vi "选择结构（成绩分类）.vi"() -> ()   [LabVIEW 2017]
panel:
  out "c成绩":string="成绩无效！！!"
  in  "分数":dbl
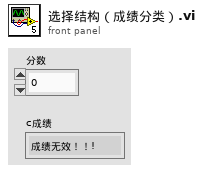
[diagram p1: front panel]
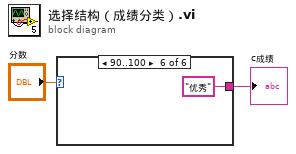
[diagram p0: block diagram]
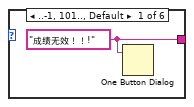
[diagram p2: hidden frame]
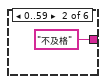
[diagram p3: hidden frame]
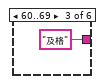
[diagram p4: hidden frame]
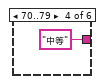
[diagram p5: hidden frame]
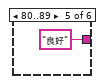
[diagram p6: hidden frame]
diagram:
  n1 = case shown="90..100" "分数" {
    tunnel: [w3 "不及格" ("消息") "及格" ("消息") "中等" ("消息") "良好" ("消息") "优秀" ("消息")] -> w1
    frame ..-1, 101.., Default {
      w3 = "成绩无效！！!" ("消息")
      n2 = One Button Dialog(message=w3) -> ()  [unwired: 1 in, 1 out]
    }
    frame 0..59 {
    }
    frame 60..69 {
    }
    frame 70..79 {
    }
    frame 80..89 {
    }
    frame 90..100 {
    }
  }
  "c成绩" <- w1
